vi "Set AGC Mode.vi"(8 "error in (no error)":errorcluster, 10 "Enable AGC (T)":bool=TRUE, 11 "device handle in":T1) -> (0 "error out":errorcluster, 3 "device handle out":T1)   [LabVIEW 2021, in "RTL-SDR.lvlib"]
uses:
  RTL-SDR.lvlib
  usr/lib64/librtlsdr.so.0
  Controls/Device Handle.ctl
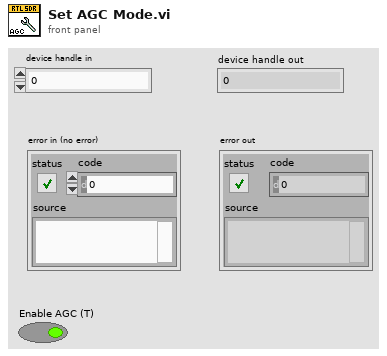
[diagram p1: front panel]
types:
  T1 = typedef "RTL-SDR.lvlib/Device Handle.ctl" = u64
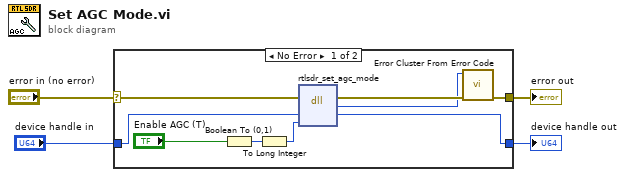
[diagram p0: block diagram]
diagram:
  n1 = case shown="No Error" "error in (no error)" {
    selector: "error in (no error)" -> [w10 w15]
    tunnel: [w12 w15] -> w4
    tunnel: "device handle in" -> [w6 w14]
    tunnel: [w5 w14] -> w1
    frame No Error {
      n2 = Boolean To (0,1)(Boolean="Enable AGC (T)") -> (0, 1=w8:i16)
      n3 = To Long Integer(number=w8) -> (32bit integer=w7:i32)
      n4 = dll-call lib="usr/lib64/librtlsdr.so.0" fn="rtlsdr_set_agc_mode"(error in=w10, "dev"=w6, "on"=w7) -> (error out=w13:errorcluster, "return type"=w11:i32, "dev"=w5:u64)  [unwired: 3 in, 1 out]
      n5 = call <vilib>:"Error Cluster From Error Code.vi"("error in (no error)"=w13, "error code (0)"=w11) -> ("error out"=w12:errorcluster)  [unwired: 7 in]
    }
    frame Error {
    }
  }
  "error out" <- w4
  "device handle out" <- w1
